vi "Create SBlock (2D params).vi"(5 "Script Path":path, 7 "Common Parameters":string[][](array[string]), 9 "Number of repetitions":u16, 11 "error in (no error)":errorcluster) -> (4 "Schedule Block out":refnum<class "Schedule Block.lvclass">, 6 "Kasli Name":string, 15 "error out":errorcluster)   [LabVIEW 2020, in "Run Utilities.lvlib" / "Schedule Block.lvclass"]
uses:
  Schedule Block.lvclass
  TALOS/TALOS_PPL.lvlibp/Support VIs/Global Memory.vi
  TALOS/TALOS_PPL.lvlibp/Interfaces/FPGA Interface/FPGA Interface.lvclass
  Schedule Block.lvclass/Schedule Block.ctl
  TALOS/TALOS_PPL.lvlibp
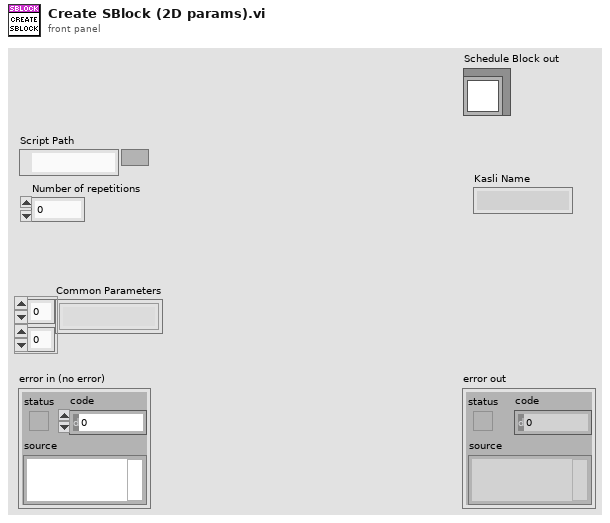
[diagram p1: front panel]
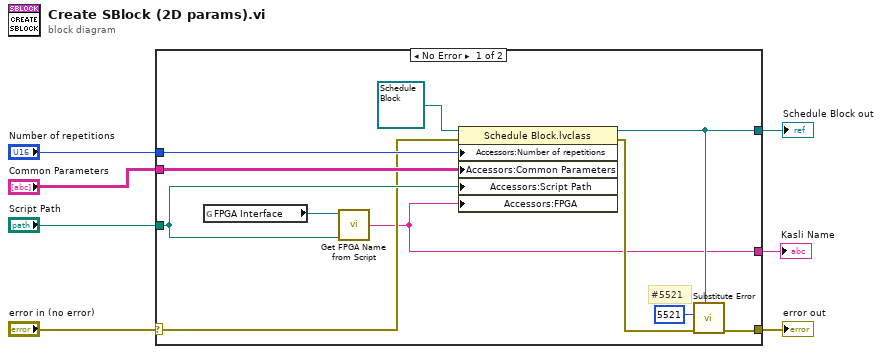
[diagram p0: block diagram]
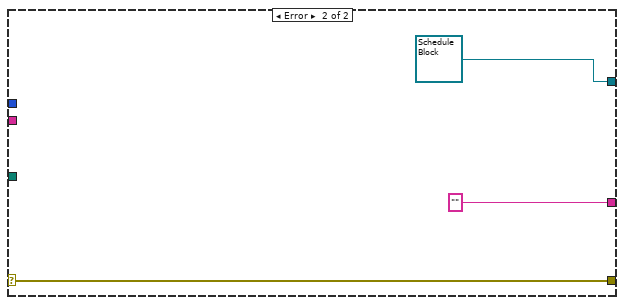
[diagram p2: hidden frame]
diagram:
  n1 = case shown="No Error" "error in (no error)" {
    selector: "error in (no error)" -> [w10 w21]
    tunnel: [w17 w21] -> w6
    tunnel: [w15 refnum<class "Schedule Block.lvclass"> refnum ("Schedule Block in")] -> w5
    tunnel: "Script Path" -> [w13 _]
    tunnel: "Number of repetitions" -> [w12 _]
    tunnel: [w9 "" ("Kasli Name")] -> w2
    tunnel: "Common Parameters" -> [w14 _]
    frame No Error {
      # "#5521"
      n2 = global read "Global Memory.vi" "FPGA Interface"() -> (w8:refnum<class "FPGA Interface.lvclass">)
      n3 = call-dynamic "Get FPGA Name from Script.vi"("file"=w13, "FPGA Interface"=w8) -> ("FPGA Name"=w9:string)  [unwired: 2 in]
      n4 = property class="Schedule Block.lvclass"(reference=refnum<class "Schedule Block.lvclass"> refnum ("Schedule Block in"), error in=w10, "Accessors:Number of repetitions"=w12, "Accessors:Common Parameters"=w14, "Accessors:Script Path"=w13, "Accessors:FPGA"=w9) -> (reference out=w15:refnum<class "Schedule Block.lvclass">, error out=w18:errorcluster)
      n5 = call "Substitute Error.vi"("LabVIEW Object"=w15, "error in (no error)"=w18, "Error Code"=5521) -> ("error out"=w17:errorcluster)  [unwired: 8 in]
    }
    frame Error {
    }
  }
  "error out" <- w6
  "Schedule Block out" <- w5
  "Kasli Name" <- w2
